vi "String_To_NumberArray_old.vi"(1 "Format":string, 2 "Input String":string) -> (0 "Output Array":dbl[](array[numeric]))   [LabVIEW 2017]
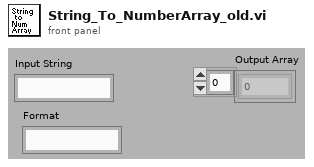
[diagram p1: front panel]
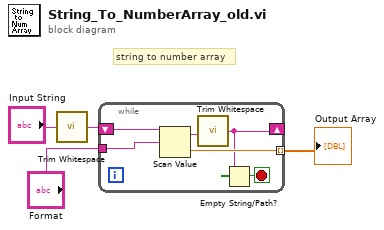
[diagram p0: block diagram]
diagram:
  # "string to number array"
  n1 = call <vilib>:"Trim Whitespace.vi"("string"="Input String") -> ("trimmed string"=w4:string)  [unwired: 1 in]
  n2 = while {
    shift-right: [w6] -> _
    shift-left: w4 -> [w8]
    tunnel: [w10] -> w1 mode=indexing
    tunnel: "Format" -> [w5]
    stop <- w7 stop-if-true
    n3 = Scan Value(string=w8, format string=w5) -> (output string=w9:string, value=w10:dbl)  [unwired: 1 out]
    n4 = call <vilib>:"Trim Whitespace.vi"("string"=w9) -> ("trimmed string"=w6:string)  [unwired: 1 in]
    n5 = Empty String/Path?(string/path=w6) -> (empty?=w7:bool)
  }
  "Output Array" <- w1
